vi "2L23_mod_expo.vi"(2 "Erreur":errorcluster caption="sortie d'erreur", 3 "t":dbl, 4 "Lambda":dbl) -> (0 "Erreur":errorcluster caption="sortie d'erreur", 1 "R(t)=exp (- Lambda * t )":dbl)   [LabVIEW 2010, in "lv_02.lvlib"]
uses:
  lv_02.lvlib
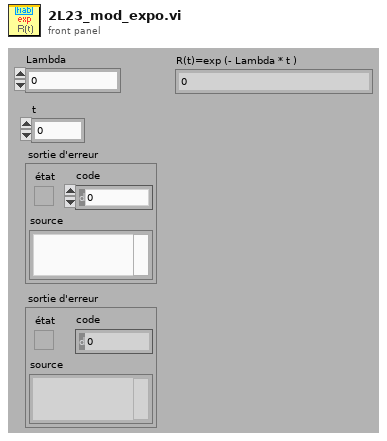
[diagram p1: front panel]
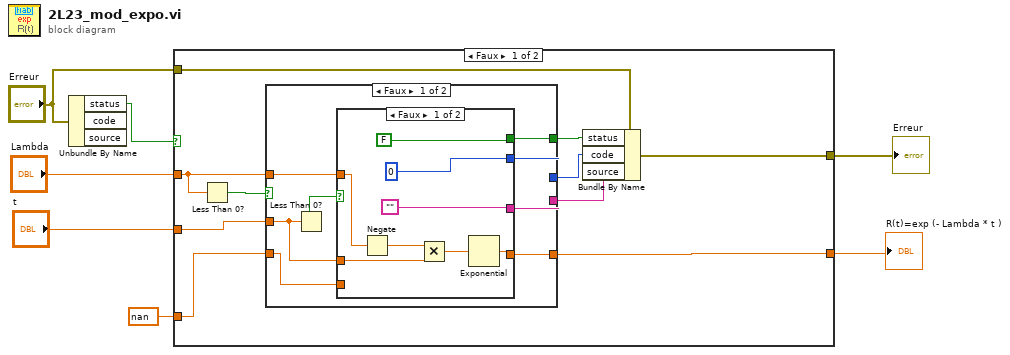
[diagram p0: block diagram]
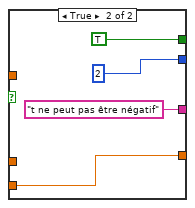
[diagram p2: hidden frame]
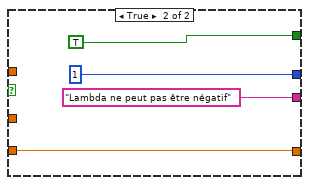
[diagram p3: hidden frame]
diagram:
  n1 = Unbundle By Name("Erreur") -> ("status"=w7:bool)  [unwired: 2 out]
  n2 = case shown="Faux" w7 {
    tunnel: "Erreur" -> [w16 w43]
    tunnel: [w15 w43] -> w5
    tunnel: "Lambda" -> [w10 _]
    tunnel: "t" -> [w11 _]
    tunnel: [w9 w42] -> w2
    tunnel: nan -> [w8 w42]
    frame False {
      n3 = Less Than 0?(x=w10) -> (x < 0?=w17:bool)
      n4 = case shown="Faux" w17 {
        tunnel: [w24 "Lambda ne peut pas être négatif"] -> w13
        tunnel: w11 -> [w21 _]
        tunnel: [w23 TRUE] -> w14
        tunnel: [w22 1] -> w12
        tunnel: w10 -> [w20 _]
        tunnel: [w19 w38] -> w9
        tunnel: w8 -> [w18 w38]
        frame False {
          n5 = Less Than 0?(x=w21) -> (x < 0?=w25:bool)
          n6 = case shown="Faux" w25 {
            tunnel: ["" "t ne peut pas être négatif"] -> w24
            tunnel: [FALSE TRUE] -> w23
            tunnel: [0 2] -> w22
            tunnel: w21 -> [w28 _]
            tunnel: w20 -> [w27 _]
            tunnel: [w26 w34] -> w19
            tunnel: w18 -> [_ w34]
            frame False {
              n7 = Negate(x=w27) -> (-x=w30:dbl)
              n8 = Multiply(x=w30, y=w28) -> (x*y=w29:dbl)
              n9 = Exponential(1:w29) -> (0:w26:dbl)
            }
            frame True {
            }
          }
        }
        frame True {
        }
      }
      n10 = Bundle By Name(cluster=w16, "status"=w14, "code"=w12, "source"=w13) -> (w15:errorcluster)
    }
    frame True {
    }
  }
  "Erreur" <- w5
  "R(t)=exp (- Lambda * t )" <- w2
